vi "WaitKick.vi"(4 "KickTarget":dbl[](array[numeric]), 5 "firstCall?":bool, 6 "target gap":dbl[](array[numeric]), 8 "error in (no error)":errorcluster, 9 "Game":refnum<class "Game.lvclass">, 10 "Robot":refnum<class "Robot.lvclass">, 11 "KickToSkill in":refnum<class "KickToSkill.lvclass">) -> (0 "error out":errorcluster, 2 "Robot out":refnum<class "Robot.lvclass">, 3 "KickToSkill out":refnum<class "KickToSkill.lvclass">)   [LabVIEW 2023, in "KickToSkill.lvclass"]
uses:
  KickToSkill.lvclass
  Robot_class/Robot.lvclass
  Game_class/Game.lvclass
  KickToSkill.lvclass/KickToSkill.ctl
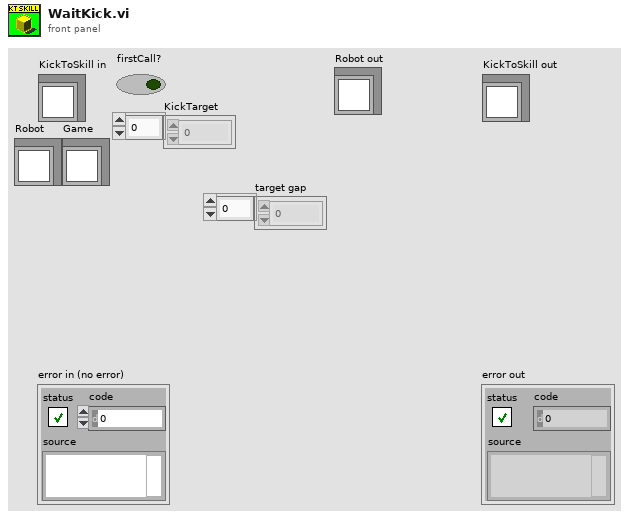
[diagram p1: front panel]
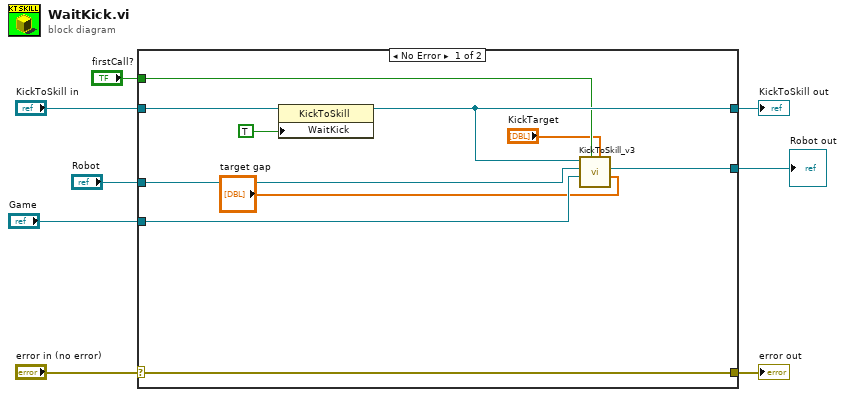
[diagram p0: block diagram]
diagram:
  n1 = case shown="No Error" "error in (no error)" {
    selector: "error in (no error)" -> [w18 w21]
    tunnel: [w18 w21] -> w7
    tunnel: [w15 w20] -> w5
    tunnel: "KickToSkill in" -> [w17 w20]
    tunnel: "Robot" -> [w14 w19]
    tunnel: "Game" -> [w13 _]
    tunnel: "firstCall?" -> [w12 _]
    tunnel: [w10 w19] -> w1
    frame No Error {
      n2 = property class="KickToSkill"(reference=w17, "WaitKick"=TRUE) -> (reference out=w15:refnum<class "KickToSkill.lvclass">)  [unwired: 1 in, 1 out]
      n3 = call "KickToSkill_v3.vi"("target gap"="target gap", "KickTarget"="KickTarget", "firstCall?"=w12, "Game"=w13, "Robot"=w14, "KickToSkill in"=w15) -> ("Robot out"=w10:refnum<class "Robot.lvclass">)  [unwired: 3 in, 2 out]
    }
    frame Error {
    }
  }
  "error out" <- w7
  "KickToSkill out" <- w5
  "Robot out" <- w1
